vi "WaveGenerator_Sample_Program.vi"(0 "System no.":i32=1 min=1 max=4 step=1, 1 "Stop refnum":refnum<vi>, 2 "Affected axis":string="1", 3 "Selection":T1, 4 "DDL":bool, 5 "error in":errorcluster, 6 "Sine Parameters:":T3={"Xo (Start)"=0, "SIN_P Parameters"={"C"=200.0, "A"=10.0, "O"=0.0}, "N (Length)"=500, "Append? (&)"=FALSE} {"N (Length)" min=0 max=1000 step=1; "SIN_P Parameters"."O" format="%.6f"; "SIN_P Parameters"."A" format="%.6f"; "SIN_P Parameters"."C" format="%.6f"}, 7 "Ramp Parameters:":T2={"Xo (Start)"=0, "RAMP Parameters"={"C"=200.0, "J"=0.0, "A"=8.0, "O"=0.0}, "N (Length)"=500, "Append? (&)"=FALSE} {"N (Length)" min=0 max=1000 step=1; "RAMP Parameters"."O" format="%.6f"; "RAMP Parameters"."A" format="%.6f"; "RAMP Parameters"."J" format="%.6f"; "RAMP Parameters"."C" format="%.6f"}, 8 "Start position":dbl format="%.6f") -> (14 "Waveform":dbl[][](graph) caption="Graph showing the commanded (green) and measured (white) waveform and the position error (red).", 19 "Error out":errorcluster)   [LabVIEW 2015]
doc: "This VI demonstrates how to use the wave generator command VIs. It first moves the affected axis to a given start position. Then it runs in a loop, giving the user the options to write sine wave curve segments or ramps into the controllers wave buffer. Wave storage data points are limited to 1000 points to keep transfer times low. The segment length of one waveform - which normally defines the frequency - is predefined as 500 points in this example. Depending on the value of Append? (&), either the old buffer data is overwritten or the new wave will be appended to memory. Please take into account that you can append at most two waveforms since buffer size is limited to 1000 points as mentioned above. \n\nAdjust the following controls to modify the shape of the waveforms.\nN (Length): Waveform (i.e. the points to be modified) goes from 1 to Length. Datapoints from Length to 500 are filled with value of last wave point.\nXo (Start): Position where the first point of the waveform is located. \nC: Center point of the wave. If C = Length/2 then the wave is symmetrical.\nA: Amplitude of the waveform. F(x) = A*sin(x) + O\nO: Offset of the waveform. F(x) = A*sin(x) + O\nJ: Jerk. Means curvature in the transition to or from standstill.\n\nYou have to stop generator output prior to restarting it with a different parameter set. The Start Gen. and Stop Gen. buttons will enable or disable the wave generator output by sending \"WGO 0\" or \"WGO 1\" for the affected axis. If DDL is enabled \"WGO 65\" will be sent respectively. The red Stop button stops the wave generator output on the specified axis and finishes the loop. Please respect the delays that occur while the controller is processing your commands. This is indicated by the \"Busy?\" indicator. See manual for further details. \n\nIn case of an error a button Clear Error will appear and the control buttons above will be disabled. Pressing this button will clear the error status and enable the control buttons again.\nWith DDL ON you can achieve significantly better position accuracy. Compare the target (green), response (white) and error (red) signals on the graph. Since this is a very sensitive mechanism we recommend starting with low amplitudes and adjusting the parameters with caution. The DDL button works only if the controller supports DDL. Contact PI for information on activation of DDL support.\n\nSee User Manual for details about the use of the wave generator.\n\nRun XXXX_Configuration_Setup (with XXXX being the product number of your PI controller) prior to running this VI.\n\nValid for: E-712, E-725, E-753"
panel:
  out "Gen. running?":bool
  out "DDL":bool
  in  "Clear Error":bool
  out "Busy?":bool
  out "Controller error":bool
  in  "Stop":bool
  # "Wave generator sample program"
  # "This VI demonstrates how to use the wave generator command VIs. It first moves the affected axis to a given start position. Then it runs in a loop, giving the\nuser the options to write sine wave curve segments or ramps into the controllers wave buffer. Wave storage data points are limited to 1000 points\nto keep transfer times low. The segment length of one waveform is predefined as 500 points in this example. Depending on the value of Append? (&), either\nthe old buffer data is overwritten or the new wave will be appended to memory. You have to stop generator output prior to restarting it with a different\nparameter set. The Start Gen. and Stop Gen. buttons will enable or disable the wave generator output by sending \"WGO 0\" or \"WGO 1\" for the affected axis. \nIf DDL is enabled \"WGO 65\" will be sent respectively. The red Stop button stops the wave generator output on the specified axis and finishes the loop. Please\nrespect the delays that occur while the controller is processing your commands. This is indicated by the \"Busy?\" indicator. See manual for further details. \nRun XXXX_Configuration_Setup (with XXXX being the product number of your PI controller) prior to running this VI."
  # "DDL state"
  # "Stop VI\nand wave\ngenerator\noutput"
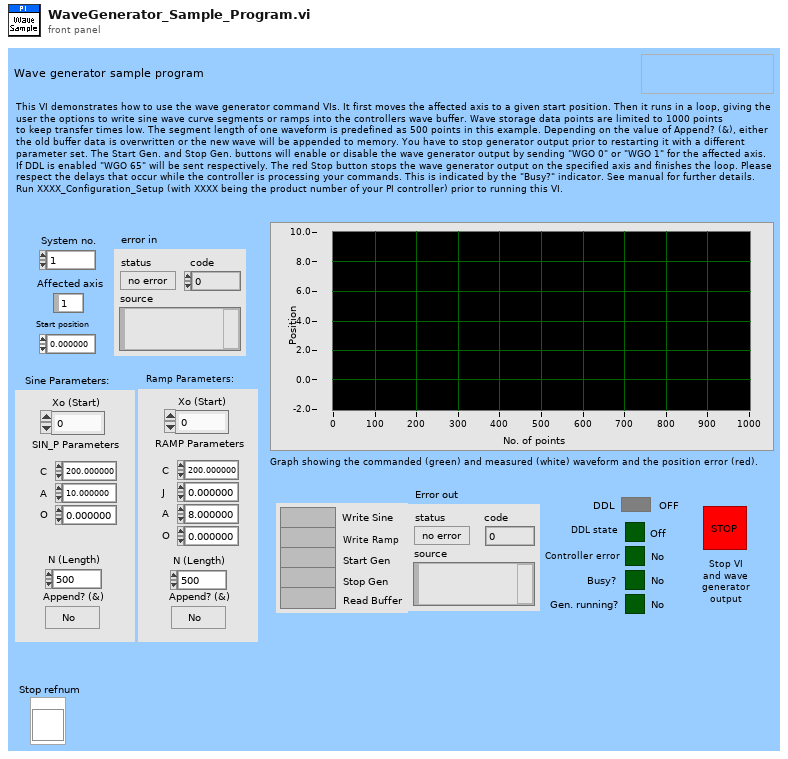
[diagram p1: front panel]
types:
  T1 = cluster{"Write Sine":bool, "Write Ramp":bool, "Start Gen":bool, "Stop Gen":bool, "Read Buffer":bool}
  T2 = cluster{"Xo (Start)":i32, "RAMP Parameters":cluster{"C":dbl, "J":dbl, "A":dbl, "O":dbl}, "N (Length)":i32, "Append? (&)":bool}
  T3 = cluster{"Xo (Start)":i32, "SIN_P Parameters":cluster{"C":dbl, "A":dbl, "O":dbl}, "N (Length)":i32, "Append? (&)":bool}
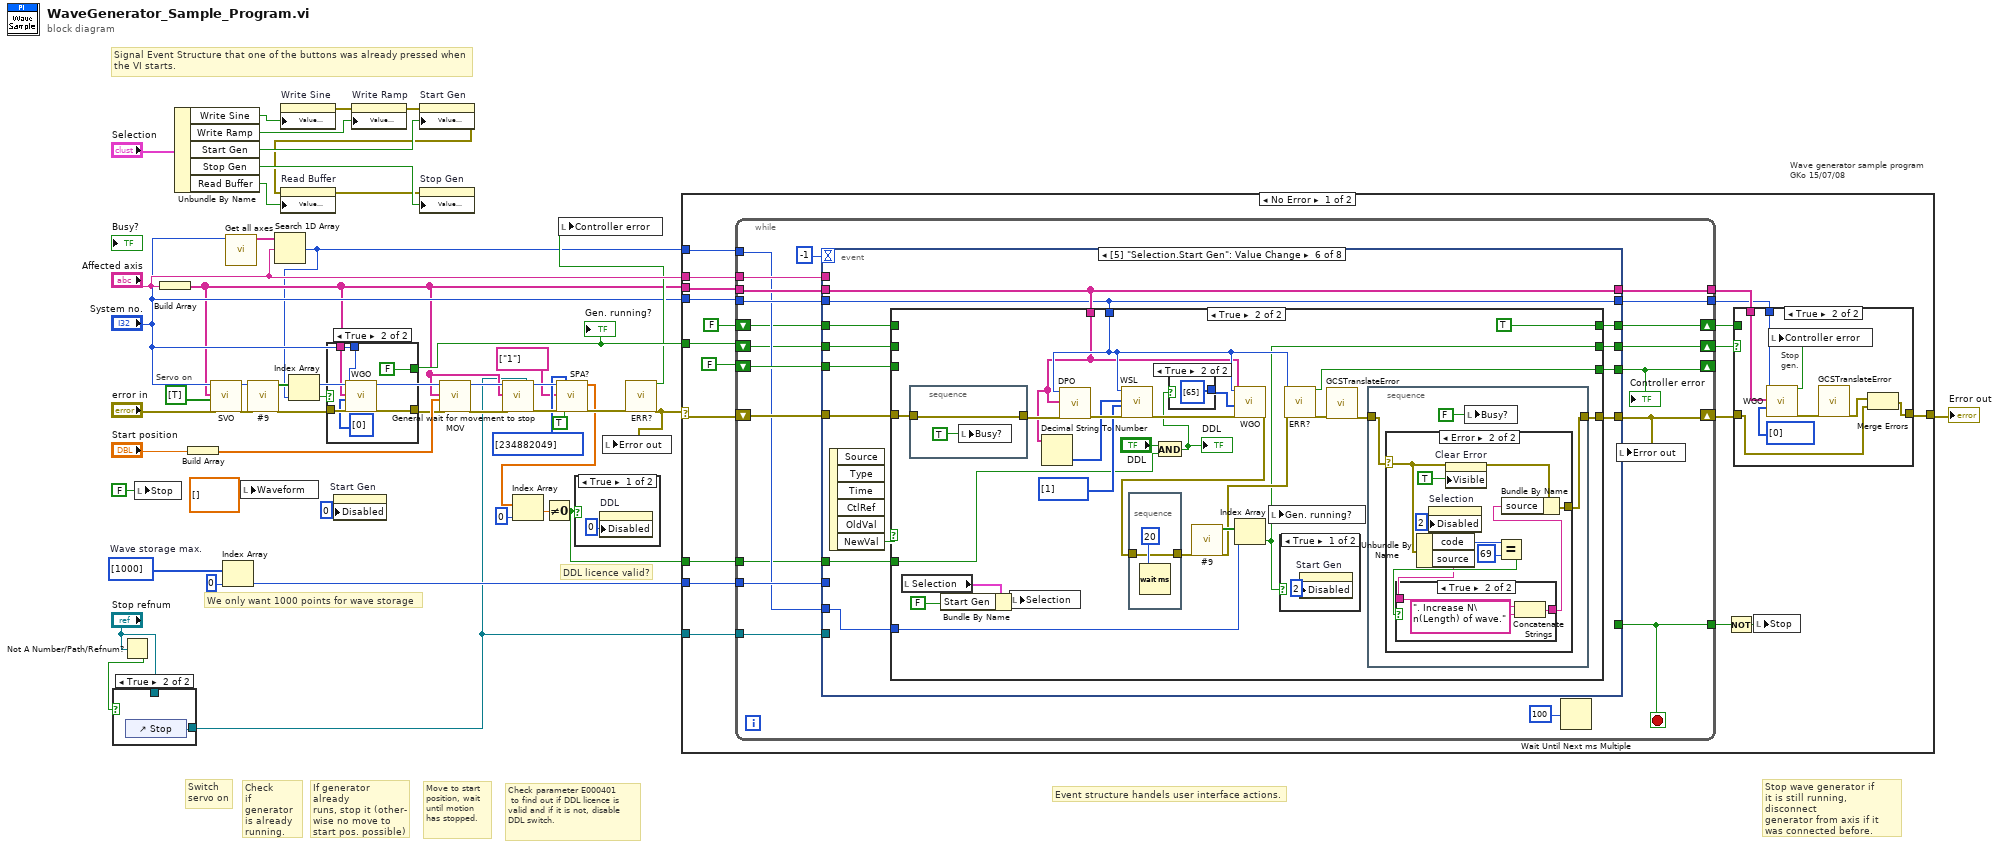
[diagram p0: block diagram]
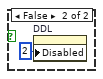
[diagram p2: hidden frame]
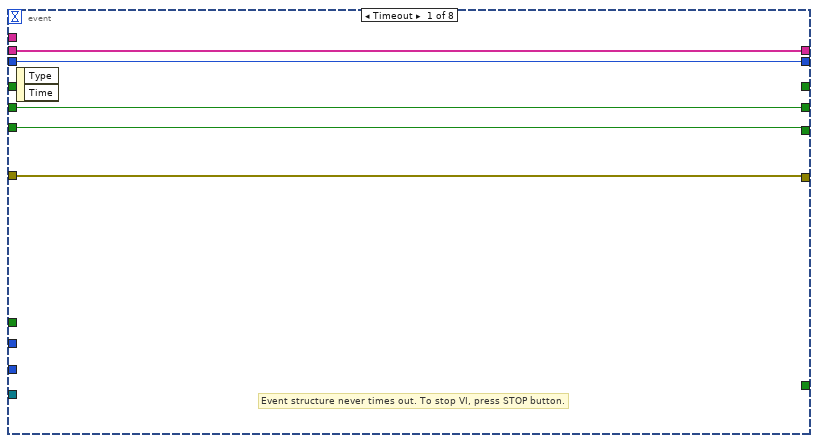
[diagram p6: hidden frame]
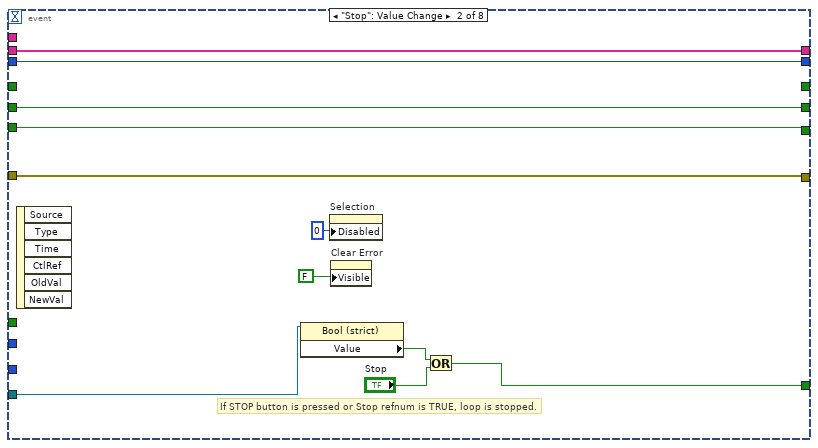
[diagram p7: hidden frame]
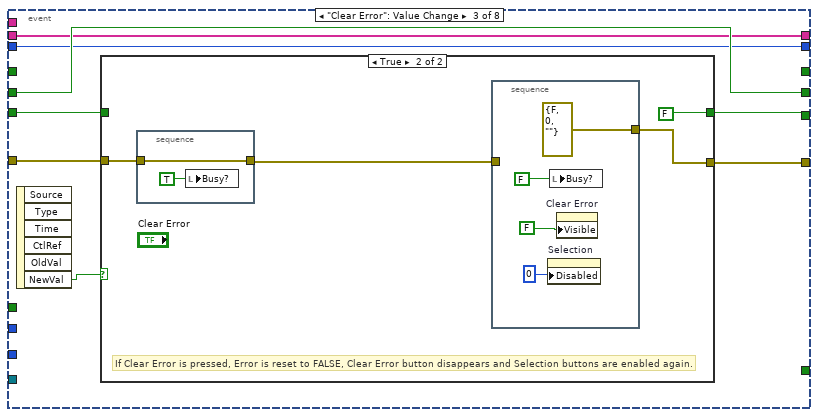
[diagram p8: hidden frame]
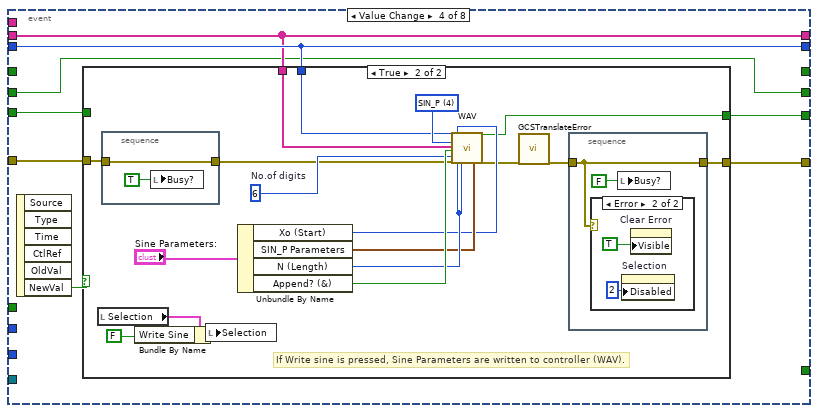
[diagram p10: hidden frame]
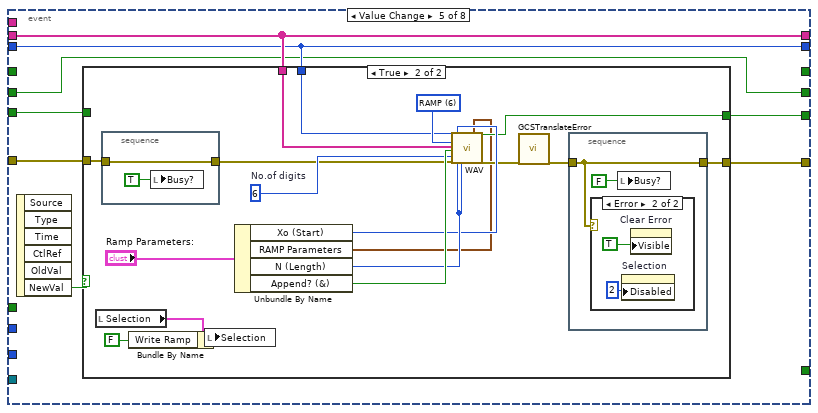
[diagram p13: hidden frame]
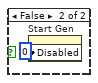
[diagram p17: hidden frame]
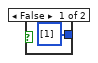
[diagram p18: hidden frame]
diagram:
  w44 = i32[] [1000]  # Wave storage max.
  # "Stop wave generator if\nit is still running, disconnect \ngenerator from axis if it\nwas connected before."
  # "Event structure handels user interface actions."
  # "Check parameter E000401\n to find out if DDL licence is\nvalid and if it is not, disable\nDDL switch."
  # "If generator already\nruns, stop it (other-\nwise no move to\nstart pos. possible)"
  # "Check\nif generator\nis already \nrunning."
  # "We only want 1000 points for wave storage"
  # "Switch\nservo on"
  # "Signal Event Structure that one of the buttons was already pressed when\nthe VI starts."
  # "DDL licence valid?"
  # "Servo on"
  # "Move to start\nposition, wait\nuntil motion\nhas stopped."
  # "Wave generator sample program\nGKo 15/07/08"
  n1 = Not A Number/Path/Refnum?(number/path/refnum="Stop refnum") -> (NaN/Path/Refnum?=w40:bool)
  n2 = case shown="True" w40 {
    tunnel: [w48 w49] -> w6
    tunnel: "Stop refnum" -> [w48 _]
    frame False {
    }
    frame True {
      n3 = control-ref of="Stop"() -> (w49:refnum<vi>)
    }
  }
  n4 = local write "Stop"(FALSE ("Controller error")) -> ()
  n5 = Build Array("Affected axis") -> (w20:string[])
  n6 = Unbundle By Name("Selection") -> ("Write Sine"=w11:bool, "Write Ramp"=w10:bool, "Start Gen"=w9:bool, "Stop Gen"=w8:bool, "Read Buffer"=w7:bool)
  n7 = Build Array("Start position") -> (w41:dbl[])
  n8 = call "SVO.vi"("System no."="System no.", "Axes to command"=w20, "Servo mode"=bool[] [TRUE], "error in"="error in") -> ("error out"=w34:errorcluster)  [unwired: 15 in]
  n9 = Index Array(array=w44, index=0 ("Index")) -> (element=w45:i32)
  n10 = call "Get all axes.vi"("System no."="System no.") -> ("Conn. Axes"=w36:string[])  [unwired: 18 in]
  n11 = local write "Waveform"(dbl[][] [] ("Waveform")) -> ()
  n12 = call "#9.vi"("System no."="System no.", "error in"=w34) -> ("WG running?"=w37:bool[], "error out"=w29:errorcluster)  [unwired: 16 in]
  n13 = Search 1D Array(1D array=w36, element="Affected axis") -> (index of element=w16:i32)  [unwired: 1 in]
  n14 = property on="Write Sine" class="Bool (strict)"("Value (Signaling)"=w11) -> (error out=w5:errorcluster)  [unwired: 2 in, 1 out]
  n15 = Index Array(array=w37, index=w16) -> (element=w30:bool)
  n16 = case shown="True" w30 {
    selector: w30 -> [w51 _]
    tunnel: w29 -> [w50 w57]
    tunnel: [w50 w56] -> w28
    tunnel: "System no." -> [_ w54]
    tunnel: w20 -> [_ w53]
    tunnel: [w51 FALSE] -> w27
    frame False {
    }
    frame True {
      n17 = call "WGO.vi"("System no."=w54, "Affected axes"=w53, "WGO Parameter"=i32[] [0], "error in"=w57) -> ("error out"=w56:errorcluster)  [unwired: 14 in, 1 out]
    }
  }
  "Gen. running?" <- w27
  n18 = property on="Start Gen" class="Bool (strict)"("Disabled"=u8 0) -> ()  [unwired: 2 in, 2 out]
  n19 = property on="Write Ramp" class="Bool (strict)"(error in=w5, "Value (Signaling)"=w10) -> (error out=w4:errorcluster)  [unwired: 1 in, 1 out]
  n20 = property on="Start Gen" class="Bool (strict)"(error in=w4, "Value (Signaling)"=w9) -> (error out=w3:errorcluster)  [unwired: 1 in, 1 out]
  n21 = property on="Stop Gen" class="Bool (strict)"(error in=w3, "Value (Signaling)"=w8) -> (error out=w2:errorcluster)  [unwired: 1 in, 1 out]
  n22 = property on="Read Buffer" class="Bool (strict)"(error in=w2, "Value (Signaling)"=w7) -> ()  [unwired: 1 in, 2 out]
  n23 = call "MOV.vi"("System no."="System no.", "Axes to move"=w20, "Position values"=w41, "error in"=w28) -> ("error out"=w31:errorcluster)  [unwired: 15 in]
  n24 = call "General wait for movement to stop.vi"("System no."="System no.", "Axes to wait for"=w20, "error in"=w31, "Stop refnum"=w6) -> ("error out"=w22:errorcluster)  [unwired: 14 in, 1 out]
  n25 = call "SPA?.vi"("System no."="System no.", "Axes to query"=string[] ["1"], "error in"=w22, "Parameter no. (hex)"=u32[] [234882049], "Parameter no. format \n(Decimal: FALSE)"=TRUE ("Parameter no. format \n(Decimal: FALSE)")) -> ("Parameter value"=w17:dbl[], "error out"=w23:errorcluster)  [unwired: 9 in, 4 out]
  n26 = Index Array(array=w17, index=0) -> (element=w14:dbl)
  n27 = Not Equal To 0?(x=w14) -> (x != 0?=w13:bool)
  n28 = case shown="True" w13 {
    frame True {
      n29 = property on="DDL" class="Bool (strict)"("Disabled"=u8 0) -> ()  [unwired: 2 in, 2 out]
    }
    frame False {
      n30 = property on="DDL" class="Bool (strict)"("Disabled"=u8 2) -> ()  [unwired: 2 in, 2 out]
    }
  }
  n31 = call "ERR?.vi"("error in"=w23) -> ("Controller error"=w25:bool, "error out"=w26:errorcluster)  [unwired: 17 in]
  n32 = local write "Controller error"(w25) -> ()
  n33 = local write "Error out"(w26) -> ()
  n34 = case shown="No Error" w26 {
    selector: w26 -> [w70 w375]
    tunnel: w20 -> [w78 _]
    tunnel: "System no." -> [w77 _]
    tunnel: [w68 w374] -> w47
    tunnel: w45 -> [w71 _]
    tunnel: "Affected axis" -> [w73 _]
    tunnel: w16 -> [w69 _]
    tunnel: w27 -> [w67 _]
    tunnel: w13 -> [w61 _]
    tunnel: w6 -> [w60 _]
    frame No Error {
      n35 = while {
        tunnel: w73 -> [w99]
        tunnel: w71 -> [w100]
        shift-left: w70 -> [w102]
        shift-right: [w101] -> w74
        tunnel: [w103] -> w75
        tunnel: [w105] -> w76
        tunnel: w77 -> [w104]
        tunnel: w78 -> [w106]
        shift-right: [w97] -> _
        shift-left: FALSE ("Controller error") -> [w96]
        tunnel: w69 -> [w95]
        shift-right: [w93] -> w66
        shift-left: w67 -> [w94]
        tunnel: [w92] -> w65
        shift-right: [w91] -> w62
        shift-left: FALSE -> [w90]
        tunnel: w61 -> [w89]
        tunnel: w60 -> [w88]
        stop <- w92 stop-if-true
        n36 = event shown="[5] \"Selection.Start Gen\": Value Change" {
          selector: _ -> [_ _ _ _ _ _ _ _]
          dyn-events: _ -> [_ _ _ _ _ _ _ _]
          timeout: -1 -> [_ _ _ _ _ _ _ _]
          tunnel: w106 -> [w110 w121 w124 w145 w180 w219 w283 w322]
          tunnel: [w110 w121 w124 w145 w180 w219 w283 w322] -> w105
          tunnel: w104 -> [w109 w120 w125 w146 w179 w218 w282 w323]
          tunnel: [w109 w120 w125 w146 w179 w218 w282 w323] -> w103
          tunnel: w102 -> [w111 w122 w127 w149 w183 w222 w287 w329]
          tunnel: [w111 w122 w128 w150 w184 w223 w288 w330] -> w101
          tunnel: w100 -> [_ _ _ _ _ _ _ w324]
          tunnel: w99 -> [_ _ _ _ _ _ _ w325]
          tunnel: [w112 w123 w129 w151 w185 w224 w289 w331] -> w97
          tunnel: w96 -> [w112 w123 w130 w147 w181 w220 w285 w327]
          tunnel: w95 -> [_ _ _ _ _ w212 w284 w326]
          tunnel: [_ w115 _ _ _ _ _ _] -> w92
          tunnel: w94 -> [w108 w119 w126 w144 w178 w216 w280 w321]
          tunnel: [w108 w119 w126 w144 w178 w217 w281 w321] -> w93
          tunnel: [_ _ _ _ _ w215 _ _] -> w91
          tunnel: w90 -> [_ _ _ _ _ w214 _ _]
          tunnel: w89 -> [_ _ _ _ _ w213 _ _]
          tunnel: w88 -> [_ w118 _ _ _ _ _ _]
          event Timeout {
            # "Event structure never times out. To stop VI, press STOP button."
            n37 = event-data() -> ()  [unwired: 1 in, 2 out]
          }
          event "Stop": Value Change {
            # "If STOP button is pressed or Stop refnum is TRUE, loop is stopped."
            n38 = event-data() -> ()  [unwired: 1 in, 6 out]
            n39 = property class="Bool (strict)"(reference=w118) -> ("Value"=w117:bool)  [unwired: 1 in, 2 out]
            n40 = property on="Selection" class="Clust (strict)"("Disabled"=u8 0) -> ()  [unwired: 2 in, 2 out]
            n41 = property on="Clear Error" class="Bool"("Visible"=FALSE) -> ()  [unwired: 2 in, 2 out]
            n42 = Or(x=w117, y="Stop") -> (x .or. y?=w115:bool)
          }
          event "Clear Error": Value Change {
            n43 = event-data() -> ("NewVal"=w131:bool)  [unwired: 1 in, 5 out]
            n44 = case shown="True" w131 {
              tunnel: w130 -> [w133 _]
              tunnel: [w133 FALSE ("Controller error")] -> w129
              tunnel: [w132 w135] -> w128
              tunnel: w127 -> [w132 w136]
              frame False {
              }
              frame True {
                # "If Clear Error is pressed, Error is reset to FALSE, Clear Error button disappears and Selection buttons are enabled again."
                n45 = stacked-sequence {
                  tunnel: w136 -> [w142]
                  tunnel: [w142] -> w134
                  frame #0 {
                    n46 = local write "Busy?"(TRUE) -> ()
                  }
                }
                n47 = stacked-sequence {
                  tunnel: [errorcluster {"status"=FALSE, "code"=0, "source"=""} ("error IO")] -> w135
                  tunnel: w134 -> [_]
                  frame #0 {
                    n48 = property on="Selection" class="Clust (strict)"("Disabled"=u8 0) -> ()  [unwired: 2 in, 2 out]
                    n49 = local write "Busy?"(FALSE) -> ()
                    n50 = property on="Clear Error" class="Bool"("Visible"=FALSE) -> ()  [unwired: 2 in, 2 out]
                  }
                }
              }
            }
          }
          event "Selection.Write Sine": Value Change {
            n51 = event-data() -> ("NewVal"=w148:bool)  [unwired: 1 in, 5 out]
            n52 = case shown="True" w148 {
              tunnel: [w152 w164] -> w151
              tunnel: w146 -> [_ w156]
              tunnel: w145 -> [_ w155]
              tunnel: [w153 w161] -> w150
              tunnel: w149 -> [w153 w160]
              tunnel: w147 -> [w152 _]
              frame False {
              }
              frame True {
                w167 = i16 6  # No.of digits
                w166 = u16 4 items=["SIN", "POL", "TAN", "PNT", "SIN_P", "LIN", "RAMP"] ("Waveform")
                # "If Write sine is pressed, Sine Parameters are written to controller (WAV)."
                n53 = local read "Selection"() -> (w159:T1)
                n54 = stacked-sequence {
                  tunnel: w160 -> [w172]
                  tunnel: [w172] -> w154
                  frame #0 {
                    n55 = local write "Busy?"(TRUE) -> ()
                  }
                }
                n56 = Bundle By Name(cluster=w159, "Write Sine"=FALSE) -> (w158:T1)
                n57 = local write "Selection"(w158) -> ()
                n58 = Unbundle By Name("Sine Parameters:") -> ("Xo (Start)"=w168:i32, "SIN_P Parameters"=w169:cluster{"C":dbl, "A":dbl, "O":dbl}, "N (Length)"=w170:i32, "Append? (&)"=w171:bool)
                n59 = call "WAV.vi"("System no."=w156, "Waveform"=w166, "Affected axes"=w155, "Append? (&)"=w171, "No.of digits"=w167, "error in"=w154, "Xo"=w168, "N"=w170, "Segment length"=w170, "SIN_P Parameters"=w169) -> ("Controller error"=w164:bool, "error out"=w163:errorcluster)  [unwired: 16 in]
                n60 = call "GCSTranslateError.vi"("error in"=w163) -> ("error out"=w162:errorcluster)  [unwired: 16 in, 2 out]
                n61 = stacked-sequence {
                  tunnel: w162 -> [w174]
                  tunnel: [w174] -> w161
                  frame #0 {
                    n62 = case shown="Error" w174 {
                      frame No Error {
                      }
                      frame Error {
                        n63 = property on="Selection" class="Clust (strict)"("Disabled"=u8 2) -> ()  [unwired: 2 in, 2 out]
                        n64 = property on="Clear Error" class="Bool"("Visible"=TRUE) -> ()  [unwired: 2 in, 2 out]
                      }
                    }
                    n65 = local write "Busy?"(FALSE) -> ()
                  }
                }
              }
            }
          }
          event "Selection.Write Ramp": Value Change {
            n66 = event-data() -> ("NewVal"=w182:bool)  [unwired: 1 in, 5 out]
            n67 = case shown="True" w182 {
              tunnel: [w186 w200] -> w185
              tunnel: w179 -> [_ w199]
              tunnel: w180 -> [_ w198]
              tunnel: [w187 w195] -> w184
              tunnel: w183 -> [w187 w194]
              tunnel: w181 -> [w186 _]
              frame False {
              }
              frame True {
                w202 = i16 6  # No.of digits
                w201 = u16 6 items=["SIN", "POL", "TAN", "PNT", "SIN_P", "LIN", "RAMP"] ("Waveform")
                n68 = local read "Selection"() -> (w190:T1)
                n69 = stacked-sequence {
                  tunnel: w194 -> [w206]
                  tunnel: [w206] -> w193
                  frame #0 {
                    n70 = local write "Busy?"(TRUE) -> ()
                  }
                }
                n71 = Bundle By Name(cluster=w190, "Write Ramp"=FALSE ("Write Sine")) -> (w189:T1)
                n72 = local write "Selection"(w189) -> ()
                n73 = Unbundle By Name("Ramp Parameters:") -> ("Xo (Start)"=w203:i32, "RAMP Parameters"=w191:cluster{"C":dbl, "J":dbl, "A":dbl, "O":dbl}, "N (Length)"=w204:i32, "Append? (&)"=w205:bool)
                n74 = call "WAV.vi"("System no."=w199, "Waveform"=w201, "Affected axes"=w198, "Append? (&)"=w205, "No.of digits"=w202, "error in"=w193, "Xo"=w203, "N"=w204, "Segment length"=w204, "RAMP Parameters"=w191) -> ("Controller error"=w200:bool, "error out"=w197:errorcluster)  [unwired: 16 in]
                n75 = call "GCSTranslateError.vi"("error in"=w197) -> ("error out"=w196:errorcluster)  [unwired: 16 in, 2 out]
                n76 = stacked-sequence {
                  tunnel: w196 -> [w208]
                  tunnel: [w208] -> w195
                  frame #0 {
                    n77 = case shown="Error" w208 {
                      frame No Error {
                      }
                      frame Error {
                        n78 = property on="Selection" class="Clust (strict)"("Disabled"=u8 2) -> ()  [unwired: 2 in, 2 out]
                        n79 = property on="Clear Error" class="Bool"("Visible"=TRUE) -> ()  [unwired: 2 in, 2 out]
                      }
                    }
                    n80 = local write "Busy?"(FALSE) -> ()
                  }
                }
              }
            }
          }
          event "Selection.Start Gen": Value Change {
            n81 = event-data() -> ("NewVal"=w221:bool)  [unwired: 1 in, 5 out]
            n82 = case shown="True" w221 {
              tunnel: [w227 w244] -> w224
              tunnel: w218 -> [_ w243]
              tunnel: w219 -> [_ w242]
              tunnel: [w228 w253] -> w223
              tunnel: w222 -> [w228 w252]
              tunnel: w220 -> [w227 _]
              tunnel: [w226 w237] -> w217
              tunnel: w216 -> [w226 _]
              tunnel: [w225 TRUE] -> w215
              tunnel: w214 -> [w225 _]
              tunnel: w213 -> [_ w231]
              tunnel: w212 -> [_ w229]
              frame False {
              }
              frame True {
                n83 = local read "Selection"() -> (w236:T1)
                n84 = stacked-sequence {
                  tunnel: w252 -> [w261]
                  tunnel: [w261] -> w246
                  frame #0 {
                    n85 = local write "Busy?"(TRUE) -> ()
                  }
                }
                n86 = Bundle By Name(cluster=w236, "Start Gen"=FALSE ("Write Sine")) -> (w235:T1)
                n87 = local write "Selection"(w235) -> ()
                n88 = Decimal String To Number(string=w242) -> (number=w247:i32[])  [unwired: 2 in, 1 out]
                n89 = call "DPO.vi"("System no."=w243, "DPO axes"=w242, "error in"=w246) -> ("error out"=w249:errorcluster)  [unwired: 16 in]
                n90 = call "WSL.vi"("System no."=w243, "Generator ID"=w247, "WaveTableID"=i32[] [1], "error in"=w249) -> ("error out"=w250:errorcluster)  [unwired: 15 in]
                n91 = And(x="DDL", y=w231) -> (x .and. y?=w230:bool)
                "DDL" <- w230
                n92 = case shown="True" w230 {
                  tunnel: [i32[] [1] ("WGO Parameter") i32[] [65] ("WGO Parameter")] -> w251
                  frame False {
                  }
                  frame True {
                  }
                }
                n93 = call "WGO.vi"("System no."=w243, "Affected axes"=w242, "WGO Parameter"=w251, "error in"=w250) -> ("error out"=w239:errorcluster)  [unwired: 14 in, 1 out]
                n94 = stacked-sequence {
                  tunnel: w239 -> [w257]
                  tunnel: [w257] -> w241
                  frame #0 {
                    n95 = Wait (ms)(milliseconds to wait=u32 20) -> ()  [unwired: 1 out]
                  }
                }
                n96 = call "#9.vi"("error in"=w241) -> ("WG running?"=w240:bool[], "error out"=w238:errorcluster)  [unwired: 17 in]
                n97 = Index Array(array=w240, index=w229) -> (element=w237:bool)
                n98 = local write "Gen. running?"(w237) -> ()
                n99 = case shown="True" w237 {
                  frame True {
                    n100 = property on="Start Gen" class="Bool (strict)"("Disabled"=u8 2) -> ()  [unwired: 2 in, 2 out]
                  }
                  frame False {
                    n101 = property on="Start Gen" class="Bool (strict)"("Disabled"=u8 0) -> ()  [unwired: 2 in, 2 out]
                  }
                }
                n102 = call "ERR?.vi"("System no."=w243, "error in"=w238) -> ("Controller error"=w244:bool, "error out"=w245:errorcluster)  [unwired: 16 in]
                n103 = call "GCSTranslateError.vi"("error in"=w245) -> ("error out"=w254:errorcluster)  [unwired: 16 in, 2 out]
                n104 = stacked-sequence {
                  tunnel: w254 -> [w264]
                  tunnel: [w263] -> w253
                  frame #0 {
                    n105 = case shown="Error" w264 {
                      selector: w264 -> [w266 w271]
                      tunnel: [w266 w269] -> w263
                      frame No Error {
                      }
                      frame Error {
                        n106 = Unbundle By Name(w271) -> ("code"=w273:i32, "source"=w267:string)
                        n107 = property on="Selection" class="Clust (strict)"("Disabled"=u8 2) -> ()  [unwired: 2 in, 2 out]
                        n108 = property on="Clear Error" class="Bool"("Visible"=TRUE) -> ()  [unwired: 2 in, 2 out]
                        n109 = Equal?(x=w273, y=69) -> (x = y?=w268:bool)
                        n110 = case shown="True" w268 {
                          tunnel: [w276 w278] -> w270
                          tunnel: w267 -> [w276 w277]
                          frame False {
                          }
                          frame True {
                            n111 = Concatenate Strings(w277, ". Increase N\n(Length) of wave.") -> (w278:string)
                          }
                        }
                        n112 = Bundle By Name(cluster=w271, "source"=w270) -> (w269:errorcluster)
                      }
                    }
                    n113 = local write "Busy?"(FALSE) -> ()
                  }
                }
              }
            }
          }
          event "Selection.Stop Gen": Value Change {
            n114 = event-data() -> ("NewVal"=w286:bool)  [unwired: 1 in, 5 out]
            n115 = case shown="True" w286 {
              tunnel: [w291 w305] -> w289
              tunnel: w282 -> [_ w299]
              tunnel: w283 -> [_ w304]
              tunnel: [w292 w309] -> w288
              tunnel: w287 -> [w292 w308]
              tunnel: w285 -> [w291 _]
              tunnel: w284 -> [_ w297]
              tunnel: [w290 w296] -> w281
              tunnel: w280 -> [w290 _]
              frame False {
              }
              frame True {
                n116 = local read "Selection"() -> (w295:T1)
                n117 = stacked-sequence {
                  tunnel: w308 -> [w315]
                  tunnel: [w315] -> w303
                  frame #0 {
                    n118 = local write "Busy?"(TRUE) -> ()
                  }
                }
                n119 = Bundle By Name(cluster=w295, "Stop Gen"=FALSE ("Write Sine")) -> (w294:T1)
                n120 = local write "Selection"(w294) -> ()
                n121 = call "WGO.vi"("System no."=w299, "Affected axes"=w304, "WGO Parameter"=i32[] [0], "error in"=w303) -> ("error out"=w302:errorcluster)  [unwired: 14 in, 1 out]
                n122 = stacked-sequence {
                  tunnel: w302 -> [w313]
                  tunnel: [w313] -> w301
                  frame #0 {
                    n123 = Wait (ms)(milliseconds to wait=u32 20) -> ()  [unwired: 1 out]
                  }
                }
                n124 = call "#9.vi"("System no."=w299, "error in"=w301) -> ("WG running?"=w298:bool[], "error out"=w300:errorcluster)  [unwired: 16 in]
                n125 = Index Array(array=w298, index=w297) -> (element=w296:bool)
                n126 = local write "Gen. running?"(w296) -> ()
                n127 = case shown="True" w296 {
                  frame True {
                    n128 = property on="Start Gen" class="Bool (strict)"("Disabled"=u8 2) -> ()  [unwired: 2 in, 2 out]
                  }
                  frame False {
                    n129 = property on="Start Gen" class="Bool (strict)"("Disabled"=u8 0) -> ()  [unwired: 2 in, 2 out]
                  }
                }
                n130 = call "ERR?.vi"("System no."=w299, "error in"=w300) -> ("Controller error"=w305:bool, "error out"=w306:errorcluster)  [unwired: 16 in]
                n131 = call "GCSTranslateError.vi"("error in"=w306) -> ("error out"=w310:errorcluster)  [unwired: 16 in, 2 out]
                n132 = stacked-sequence {
                  tunnel: w310 -> [w317]
                  tunnel: [w317] -> w309
                  frame #0 {
                    n133 = case shown="Error" w317 {
                      frame No Error {
                      }
                      frame Error {
                        n134 = property on="Selection" class="Clust (strict)"("Disabled"=u8 2) -> ()  [unwired: 2 in, 2 out]
                        n135 = property on="Clear Error" class="Bool"("Visible"=TRUE) -> ()  [unwired: 2 in, 2 out]
                      }
                    }
                    n136 = local write "Busy?"(FALSE) -> ()
                  }
                }
              }
            }
          }
          event "Selection.Read Buffer": Value Change {
            n137 = event-data() -> ("NewVal"=w328:bool)  [unwired: 1 in, 5 out]
            n138 = case shown="True" w328 {
              tunnel: [w332 w343] -> w331
              tunnel: w323 -> [_ w340]
              tunnel: w322 -> [_ _]
              tunnel: [w333 w366] -> w330
              tunnel: w329 -> [w333 w365]
              tunnel: w327 -> [w332 _]
              tunnel: w326 -> [_ _]
              tunnel: w325 -> [_ w339]
              tunnel: w324 -> [_ w337]
              frame False {
              }
              frame True {
                w351 = 3 ("Numeric")
                w352 = 2 ("Numeric")
                w359 = 1 ("Numeric")
                # "Record and display values"
                n139 = stacked-sequence {
                  tunnel: w365 -> [w368]
                  tunnel: [w368] -> w341
                  frame #0 {
                    n140 = local write "Busy?"(TRUE) -> ()
                  }
                }
                n141 = call "DRC.vi"("System no."=w340, "Rec. table"=w359, "Rec. option"=w359, "error in"=w341, "Source ID"=w339) -> ("Controller error"=w349:bool, "error out"=w358:errorcluster)  [unwired: 13 in]
                n142 = call "DRC.vi"("System no."=w340, "Rec. table"=w352, "Rec. option"=w352, "error in"=w358, "Source ID"=w339) -> ("Controller error"=w348:bool, "error out"=w357:errorcluster)  [unwired: 13 in]
                n143 = call "DRC.vi"("System no."=w340, "Rec. table"=w351, "Rec. option"=w351, "error in"=w357, "Source ID"=w339) -> ("Controller error"=w347:bool, "error out"=w350:errorcluster)  [unwired: 13 in]
                n144 = call "WGR.vi"("System no."=w340, "error in"=w350) -> ("error out"=w345:errorcluster)  [unwired: 17 in]
                n145 = call "DRR?.vi"("System no."=w340, "Rec. table IDs"=i32[] [1, 2, 3], "error in"=w345, "Xo"=1, "N"=w337, "Nmax"=w337) -> ("Data"=w362:dbl[][], "error out"=w342:errorcluster)  [unwired: 10 in, 2 out]
                n146 = Index Array(array=w362, index (col) #1=0 ("Disabled Index (col)"), index (col) #2=1 ("Disabled Index (col)"), index (col) #3=2 ("Disabled Index (col)")) -> (element #1=w360:dbl[], element #2=w354:dbl[], element #3=w353:dbl[])  [unwired: 3 in]
                n147 = Build Array(w360, w354, w353) -> (→"Waveform":dbl[][])
                n148 = call "ERR?.vi"("System no."=w340, "error in"=w342) -> ("Controller error"=w344:bool, "error out"=w364:errorcluster)  [unwired: 16 in]
                n149 = call "GCSTranslateError.vi"("error in"=w364) -> ("error out"=w367:errorcluster)  [unwired: 16 in, 2 out]
                n150 = Compound Arithmetic op=OR(w344, w349, w348, w347) -> (w343:bool)
                n151 = local read "Selection"() -> (w336:T1)
                n152 = stacked-sequence {
                  tunnel: w367 -> [w370]
                  tunnel: [w370] -> w366
                  frame #0 {
                    n153 = case shown="Error" w370 {
                      frame No Error {
                      }
                      frame Error {
                        n154 = property on="Selection" class="Clust (strict)"("Disabled"=u8 2) -> ()  [unwired: 2 in, 2 out]
                        n155 = property on="Clear Error" class="Bool"("Visible"=TRUE) -> ()  [unwired: 2 in, 2 out]
                      }
                    }
                    n156 = local write "Busy?"(FALSE) -> ()
                  }
                }
                n157 = Bundle By Name(cluster=w336, "Read Buffer"=FALSE ("Write Sine")) -> (w335:T1)
                n158 = local write "Selection"(w335) -> ()
              }
            }
          }
        }
        "Controller error" <- w97
        n159 = Wait Until Next ms Multiple(millisecond multiple=u32 100) -> ()  [unwired: 1 out]
        n160 = local write "Error out"(w101) -> ()
      }
      n161 = Not(x=w65) -> (.not. x?=w64:bool)
      n162 = case shown="True" w66 {
        tunnel: w76 -> [_ w84]
        tunnel: w75 -> [_ w85]
        tunnel: w74 -> [w79 w81]
        tunnel: [w79 w83] -> w68
        tunnel: w62 -> [_ _]
        frame False {
        }
        frame True {
          # "Stop\ngen."
          n163 = call "WGO.vi"("System no."=w85, "Affected axes"=w84, "WGO Parameter"=i32[] [0] ("WGO \nParameter")) -> ("Controller error"=w86:bool, "error out"=w80:errorcluster)  [unwired: 15 in]
          n164 = local write "Controller error"(w86) -> ()
          n165 = call "GCSTranslateError.vi"("error in"=w80) -> ("error out"=w82:errorcluster)  [unwired: 16 in, 2 out]
          n166 = Merge Errors(w82, w81) -> (w83:errorcluster)
        }
      }
      n167 = local write "Stop"(w64) -> ()
    }
    frame Error {
      n168 = call "GCSTranslateError.vi"("error in"=w375) -> ("error out"=w374:errorcluster)  [unwired: 16 in, 2 out]
    }
  }
  "Error out" <- w47
